vi "endEventToString.vi"(8 "error in (no error)":errorcluster, 11 "RampToneAmplitudeUp in":refnum<class "RampToneAmplitudeUp.lvclass">) -> (0 "error out":errorcluster, 2 "eventStringArray":string[](array[string]), 3 "RampToneAmplitudeUp out":refnum<class "RampToneAmplitudeUp.lvclass">)   [LabVIEW 2011, in "Tools.lvlib" / "Scripting.lvlib" / "RampToneAmplitudeUp.lvclass"]
uses:
  RampToneAmplitudeUp.lvclass
  SingleTone/SingleTone.lvclass
  RampTone/RampTone.lvclass
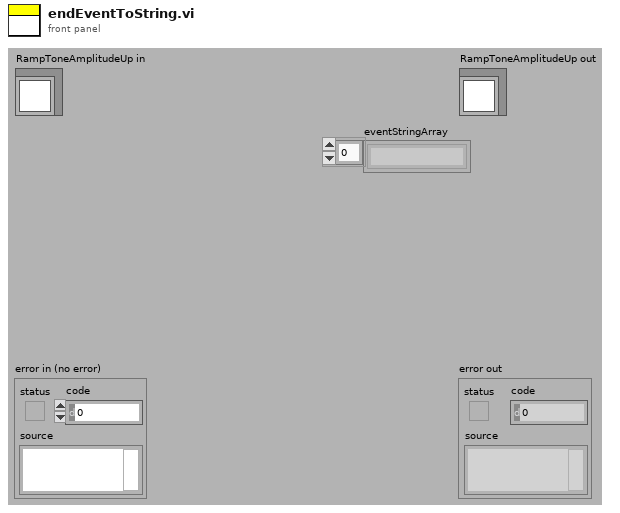
[diagram p1: front panel]
types:
  T1 = cluster{"rampTime":dbl, "timeStep":dbl, "dataValueStep":dbl}
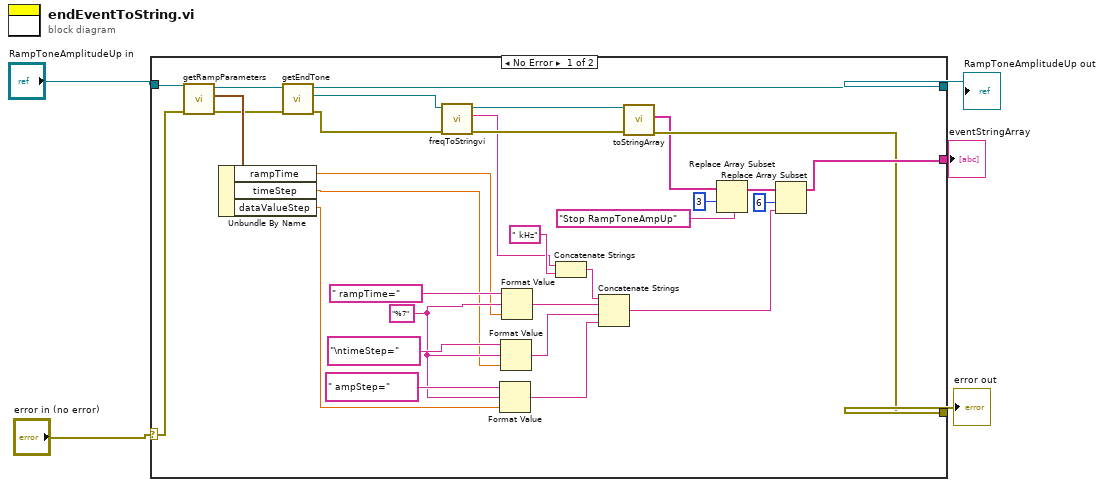
[diagram p0: block diagram]
diagram:
  n1 = case shown="No Error" "error in (no error)" {
    selector: "error in (no error)" -> [w6 w37]
    tunnel: [w21 w37] -> w2
    tunnel: [w26 _] -> w1
    tunnel: "RampToneAmplitudeUp in" -> [w16 w38]
    tunnel: [w7 w38] -> w3
    frame No Error {
      w25 = "%7"
      n2 = call "getRampParameters.vi"("error in (no error)"=w6, "RampTone in"=w16) -> ("error out"=w10:errorcluster, "RampParameters"=w15:T1, "RampTone out"=w11:refnum<class "RampToneAmplitudeUp.lvclass">)  [unwired: 7 in]
      n3 = Unbundle By Name(w15) -> ("rampTime"=w14:dbl, "timeStep"=w13:dbl, "dataValueStep"=w12:dbl)
      n4 = call-dynamic "getEndTone.vi"("error in (no error)"=w10, "RampTone.lvclass in"=w11) -> ("error out"=w9:errorcluster, "endTone.lvclass"=w8:refnum<class "SingleTone.lvclass">, "RampTone.lvclass out"=w7:refnum<class "RampToneAmplitudeUp.lvclass">)  [unwired: 7 in]
      n5 = call-dynamic "freqToStringvi.vi"("error in (no error)"=w9, "SingleTone in"=w8) -> ("error out"=w22:errorcluster, "frequency"=w18:string, "SingleTone out"=w17:refnum<class "SingleTone.lvclass">)  [unwired: 7 in]
      n6 = Format Value(string ("")=" ampStep=", format string=w25, value (0)=w12) -> (output string=w23:string)
      n7 = Format Value(string ("")="\ntimeStep=", format string=w25, value (0)=w13) -> (output string=w28:string)
      n8 = Format Value(string ("")=" rampTime=", format string=w25, value (0)=w14) -> (output string=w29:string)
      n9 = Concatenate Strings(w18, " kHz") -> (w24:string)
      n10 = Concatenate Strings(w24, w29, w28, w23) -> (w27:string)
      n11 = call-dynamic "toStringArray.vi"("error in (no error)"=w22, "SingleTone in"=w17) -> ("error out"=w21:errorcluster, "eventStringArray"=w20:string[])  [unwired: 7 in, 1 out]
      n12 = Replace Array Subset(array=w20, new element="Stop RampToneAmpUp", index=3) -> (w32:string[])
      n13 = Replace Array Subset(array=w32, new element=w27, index=6) -> (w26:string[])
    }
    frame Error {
    }
  }
  "error out" <- w2
  "RampToneAmplitudeUp out" <- w3
  "eventStringArray" <- w1
